vi "Predictor.vi"(9 "Measurement Cluster":T1, 10 "Peak Max Threshold":dbl=0.1 format="%#_13g", 11 "Data Cluster in":T3 {"Julabo Serial Configuration"."Flow Control" items=["None", "XON/XOFF", "RTS/CTS", "XON/XOFF & RTS/CTS", "DTR/DSR", "XON/XOFF & DTR/DSR"]; "Julabo Serial Configuration"."Stop Bits" items=["1.0"=10, "1.5"=15, "2.0"=20]; "Julabo Serial Configuration"."Data Bits" items=["7"=7, "8"=8]; "Julabo Serial Configuration"."Parity" items=["None", "Odd", "Even", "Mark", "Space"]; "Julabo Serial Configuration"."Baud Rate" items=["300"=300, "600"=600, "1200"=1200, "2400"=2400, "4800"=4800, "9600"=9600, "19200"=19200]; "XpU (0.6K) Ext" min=0.1 max=99.9; "Tv (0s) Ext" max=999; "Tn (3s) Ext" min=3 max=9999; "Xp (0.6K) Ext" min=0.1 max=99.9; "Tv (0s) Int" max=999; "Tn (3s) Int" min=3 max=9999; "Xp (0.6K) Int" min=0.1 max=99.9; "Lower Bandlimit" min=0.0 max=200.0; "Upper Bandlimit" min=0.0 max=200.0; "InternMin" format="%.2f"; "InternMax" format="%.2f"; "CoolMax" min=-100 max=0; "HeatMax" max=100; "Subtemp" format="%.2f"; "Overtemp" format="%.2f"; "Julabo Setpoint" format="%.2f"; "Current DoE" format="%0.3f"}) -> (3 "Data Cluster out":T3 {"Julabo Serial Configuration"."Flow Control" items=["None", "XON/XOFF", "RTS/CTS", "XON/XOFF & RTS/CTS", "DTR/DSR", "XON/XOFF & DTR/DSR"]; "Julabo Serial Configuration"."Stop Bits" items=["1.0"=10, "1.5"=15, "2.0"=20]; "Julabo Serial Configuration"."Data Bits" items=["7"=7, "8"=8]; "Julabo Serial Configuration"."Parity" items=["None", "Odd", "Even", "Mark", "Space"]; "Julabo Serial Configuration"."Baud Rate" items=["300"=300, "600"=600, "1200"=1200, "2400"=2400, "4800"=4800, "9600"=9600, "19200"=19200]; "XpU (0.6K) Ext" min=0.1 max=99.9; "Tv (0s) Ext" max=999; "Tn (3s) Ext" min=3 max=9999; "Xp (0.6K) Ext" min=0.1 max=99.9; "Tv (0s) Int" max=999; "Tn (3s) Int" min=3 max=9999; "Xp (0.6K) Int" min=0.1 max=99.9; "Lower Bandlimit" min=0.0 max=200.0; "Upper Bandlimit" min=0.0 max=200.0; "InternMin" format="%.2f"; "InternMax" format="%.2f"; "CoolMax" min=-100 max=0; "HeatMax" max=100; "Subtemp" format="%.2f"; "Overtemp" format="%.2f"; "Julabo Setpoint" format="%.2f"; "Current DoE" format="%0.3f"})   [LabVIEW 2015]
uses:
  --Controls and TypeDefs--/DoE_Control_Cluster.ctl
  <instrlib>/JULABO DeviceDriver/Examples/Julabo Serial Control.ctl
  --Controls and TypeDefs--/Measurement_Cluster.ctl
  --Controls and TypeDefs--/Raman_Model_Data_Cluster.ctl
panel:
  # "Flow Rate Measurements"
  # "Temp Measurements"
  # "Raman Measurements"
  # "Julabo"
  # "Limits"
  # "PID Control Parameters"
  # "Julabo"
  # "Limits"
  # "PID Control Parameters"
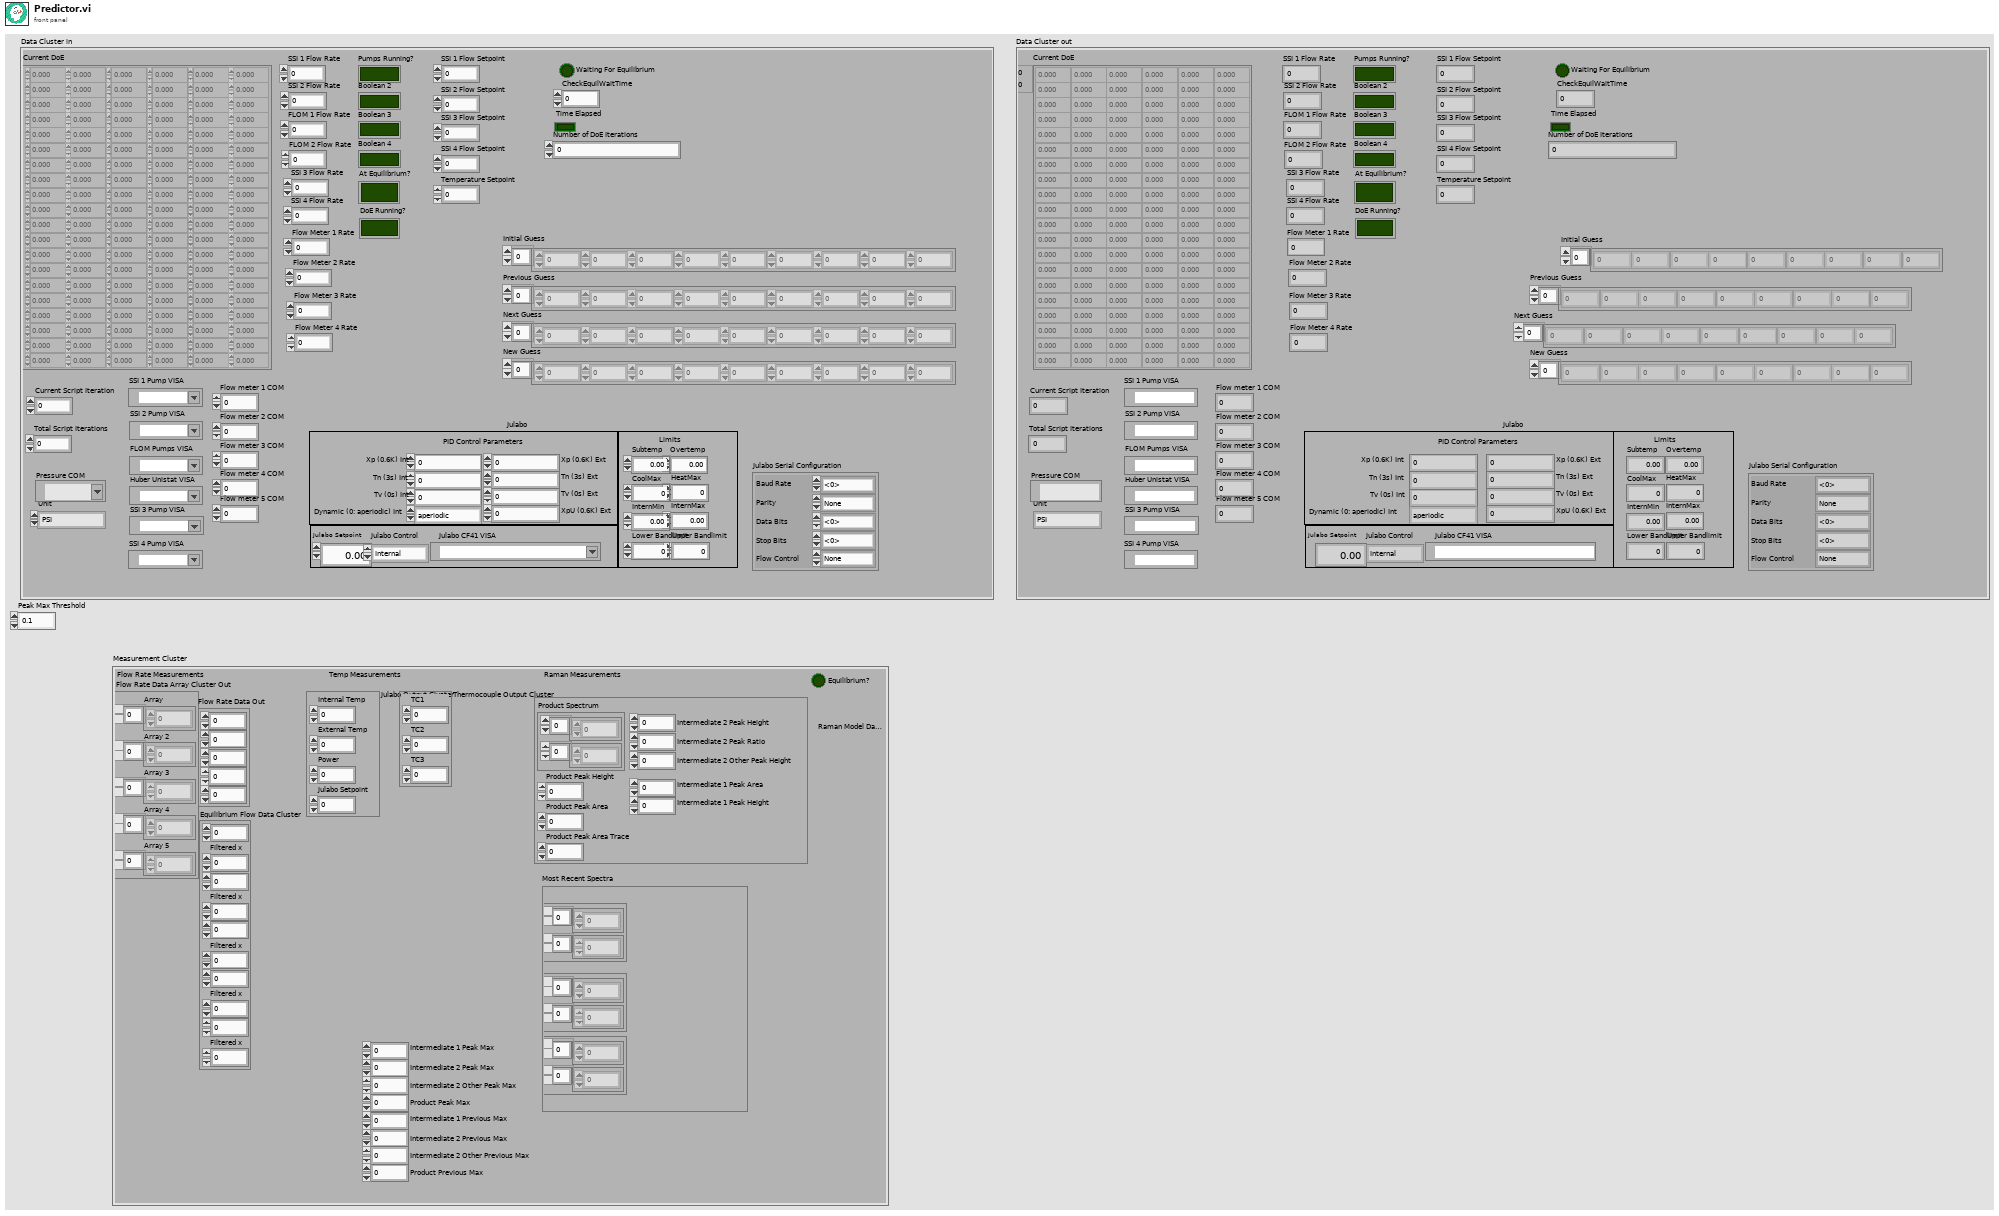
[diagram p1: front panel]
types:
  T1 = typedef "Measurement_Cluster.ctl" = cluster{"Raman Model Data Cluster":T2, "Julabo Output Cluster":cluster{"Internal Temp":dbl, "External Temp":dbl, "Power":i8, "Julabo Setpoint":dbl}, "Thermocouple Output Cluster":cluster{"TC1":dbl, "TC2":dbl, "TC3":dbl}, "Flow Rate Data Array Cluster Out":cluster{"Array":dbl[], "Array 2":dbl[], "Array 3":dbl[], "Array 4":dbl[], "Array 5":dbl[]}, "Flow Rate Data Out":cluster{dbl, dbl, dbl, dbl, dbl}, "Equilibrium?":bool, "Equilibrium Flow Data Cluster":cluster{dbl, "Filtered x":dbl, dbl, "Filtered x":dbl, dbl, "Filtered x":dbl, dbl, "Filtered x":dbl, dbl, "Filtered x":dbl}, "Most Recent Spectra":cluster{"Most recent Channel 3 (Intermediate 1) Spectrum":cluster{i32[], i32[]}, "Most recent Channel 2 (Intermediate 2) Spectrum":cluster{i32[], i32[]}, "Most recent Channel 1 (Product) Spectrum":cluster{i32[], i32[]}}, "Intermediate 2 Other Peak Max":i32, "Intermediate 2 Peak Max":i32, "Intermediate 1 Peak Max":i32, "Product Peak Max":i32, "Intermediate 2 Other Previous Max":i32, "Intermediate 2 Previous Max":i32, "Intermediate 1 Previous Max":i32, "Product Previous Max":i32}
  T2 = typedef "Raman_Model_Data_Cluster.ctl" = cluster{"Product Spectrum":cluster{i32[], i32[]}, "Product Peak Height":i32, "Product Peak Area":i32, "Product Peak Area Trace":i32, "Intermediate 2 Peak Height":i32, "Intermediate 1 Peak Area":i32, "Intermediate 1 Peak Height":i32, "Intermediate 2 Other Peak Height":i32, "Intermediate 2 Peak Ratio":i32}
  T3 = typedef "DoE_Control_Cluster.ctl" = cluster{"Current DoE":dbl[][], "SSI 1 Flow Rate":dbl, "SSI 2 Flow Rate":dbl, "FLOM 1 Flow Rate":dbl, "FLOM 2 Flow Rate":dbl, "Pumps Running?":bool, "Boolean 2":bool, "Boolean 3":bool, "Boolean 4":bool, "At Equilibrium?":bool, "DoE Running?":bool, "Current Script Iteration":dbl, "Total Script Iterations":dbl, "FLOM Pumps VISA":refnum<visa-resource-name>, "SSI 1 Pump VISA":refnum<visa-resource-name>, "SSI 2 Pump VISA":refnum<visa-resource-name>, "Huber Unistat VISA":refnum<visa-resource-name>, "SSI 3 Pump VISA":refnum<visa-resource-name>, "SSI 4 Pump VISA":refnum<visa-resource-name>, "SSI 4 Flow Rate":dbl, "SSI 3 Flow Rate":dbl, "Flow Meter 1 Rate ":dbl, "Flow Meter 2 Rate":dbl, "Flow Meter 3 Rate":dbl, "Flow Meter 4 Rate":dbl, "SSI 1 Flow Setpoint":dbl, "SSI 2 Flow Setpoint":dbl, "SSI 3 Flow Setpoint":dbl, "SSI 4 Flow Setpoint":dbl, "Temperature Setpoint":dbl, "Flow meter 3 COM":u16, "Flow meter 5 COM":u16, "Flow meter 4 COM":u16, "Flow meter 2 COM":u16, "Flow meter 1 COM":u16, "Unit":enum16{"PSI", "Bar", "cm H2O", "ft H2O", "hectoPascal", "in Hg", "in H2O", "kiloPascal", "milliBar", "mmHg", "MegaPascal", "Numeric Pressure"}, "Pressure COM":refnum<visa-resource-name>, "Julabo Setpoint":dbl, "Julabo Control":enum16{"Internal", "External"}, "Overtemp":dbl, "Subtemp":dbl, "HeatMax":u8, "CoolMax":i8, "InternMax":dbl, "InternMin":dbl, "Upper Bandlimit":dbl, "Lower Bandlimit":dbl, "Julabo CF41 VISA":refnum<visa-resource-name>, "Xp (0.6K) Int":dbl, "Tn (3s) Int":u16, "Tv (0s) Int":u16, "Dynamic (0: aperiodic) Int":enum16{"aperiodic", "standard"}, "Xp (0.6K) Ext":dbl, "Tn (3s) Ext":u16, "Tv (0s) Ext":u16, "XpU (0.6K) Ext":dbl, "Julabo Serial Configuration":T4, "Waiting For Equilibrium":bool, "CheckEquilWaitTime":dbl, "Time Elapsed":bool, "Initial Guess":dbl[], "Next Guess":dbl[], "Previous Guess":dbl[], "Number of DoE Iterations":i32, "New Guess":dbl[]}
  T4 = typedef "Julabo Serial Control.ctl" = cluster{"Baud Rate":u32, "Parity":u16, "Data Bits":u16, "Stop Bits":u16, "Flow Control":u16}
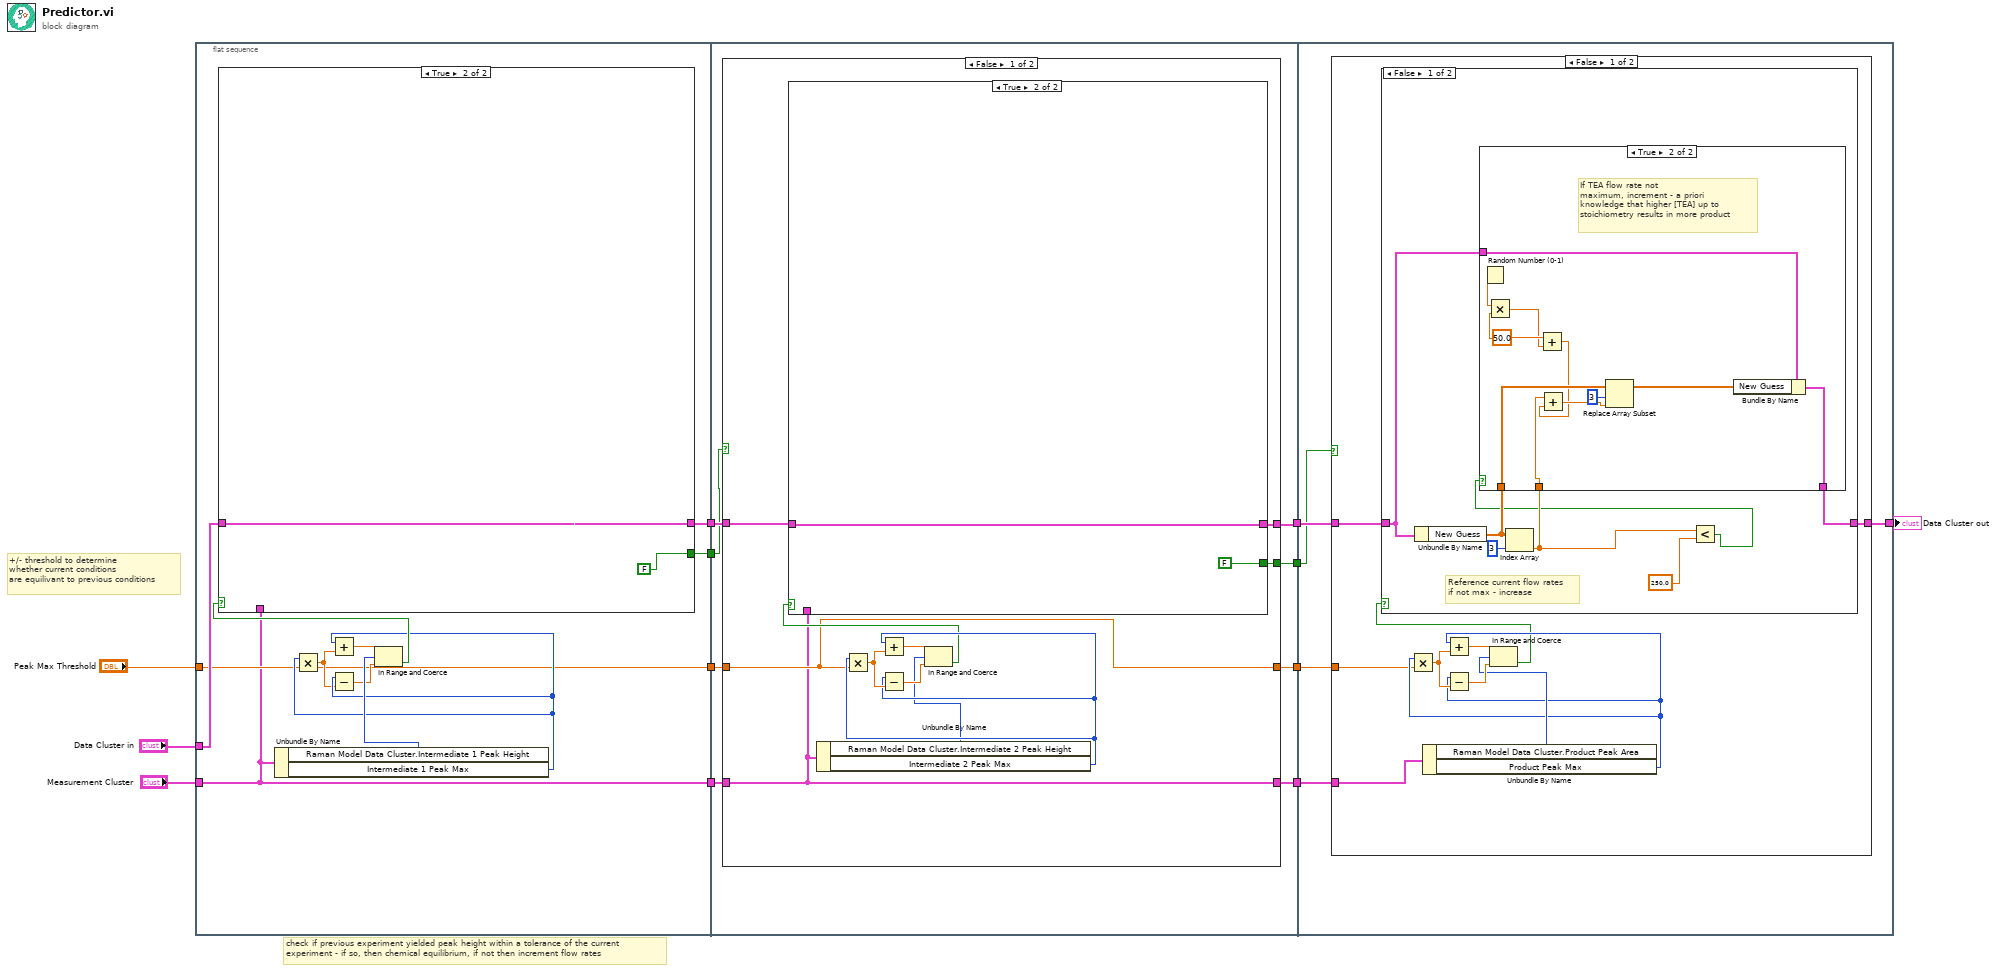
[diagram p0: block diagram]
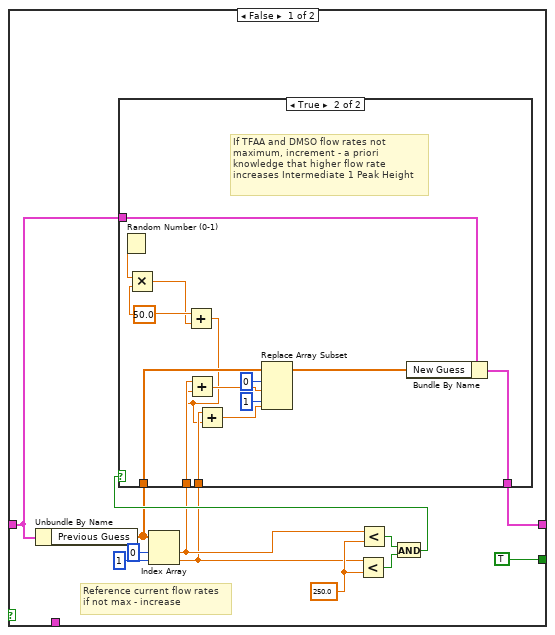
[diagram p2: hidden frame]
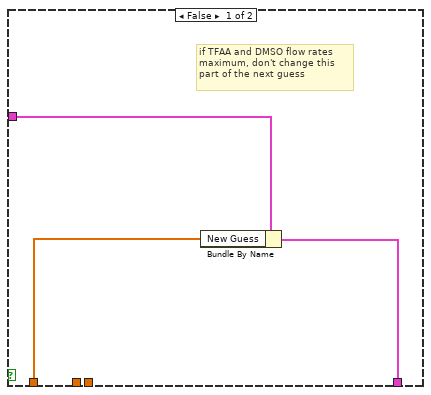
[diagram p3: hidden frame]
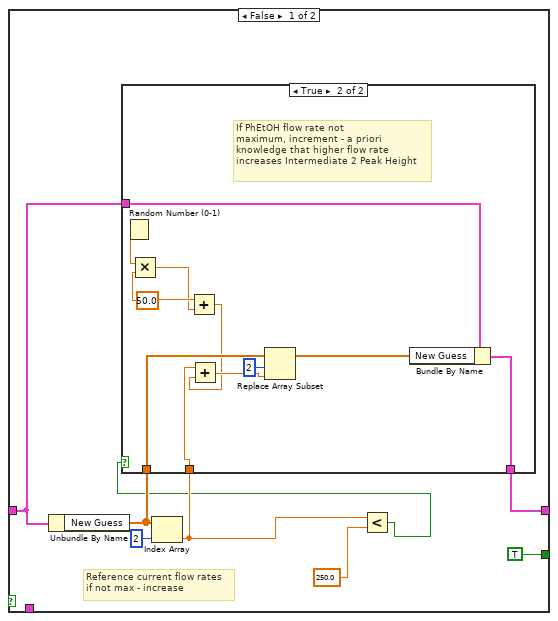
[diagram p4: hidden frame]
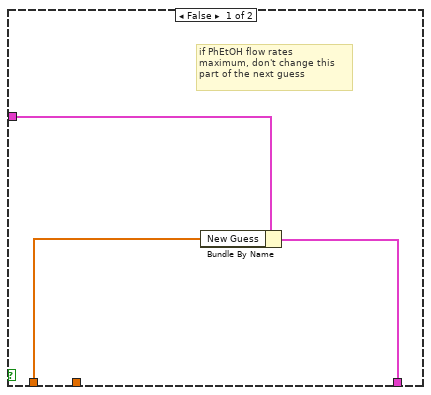
[diagram p5: hidden frame]
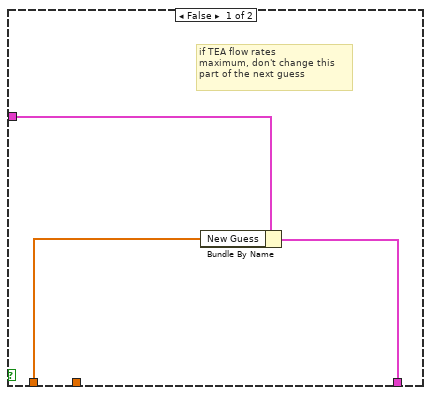
[diagram p7: hidden frame]
diagram:
  # "check if previous experiment yielded peak height within a tolerance of the current\nexperiment - if so, then chemical equilibrium, if not then increment flow rates"
  # "+/- threshold to determine\nwhether current conditions\nare equilivant to previous conditions"
  n1 = flat-sequence {
    tunnel: [w23] -> w12
    tunnel: "Data Cluster in" -> [w21]
    tunnel: "Measurement Cluster" -> [w14]
    tunnel: [w14] -> w7
    tunnel: "Peak Max Threshold" -> [w15]
    tunnel: [w15] -> w4
    tunnel: [w13] -> w3
    tunnel: w12 -> [w61]
    tunnel: [w59] -> w11
    tunnel: w7 -> [w60]
    tunnel: [w57] -> w6
    tunnel: w4 -> [w62]
    tunnel: w3 -> [w56]
    tunnel: [w58] -> w2
    tunnel: [w55] -> w1
    tunnel: w11 -> [w104]
    tunnel: [w103] -> w10
    tunnel: w6 -> [w105]
    tunnel: w2 -> [w106]
    tunnel: w1 -> [w102]
    frame #0 {
      n2 = Unbundle By Name(w14) -> ("Raman Model Data Cluster.Intermediate 1 Peak Height"=w20:i32, "Intermediate 1 Peak Max"=w19:i32)
      n3 = Multiply(x=w19, y=w15) -> (x*y=w18:dbl)
      n4 = Add(x=w19, y=w18) -> (x+y=w17:dbl)
      n5 = Subtract(x=w19, y=w18) -> (x-y=w16:dbl)
      n6 = In Range and Coerce(upper limit=w17, x=w20, lower limit=w16) -> (In Range?=w22:bool)  [unwired: 1 out]
      n7 = case shown="True" w22 {
        tunnel: [w25 w54] -> w23
        tunnel: w21 -> [w29 w54]
        tunnel: w14 -> [_ _]
        tunnel: [TRUE FALSE] -> w13
        frame False {
          w32 = 250.0 ("y")
          # "Reference current flow rates\nif not max - increase"
          n8 = Unbundle By Name(w29) -> ("Previous Guess"=w28:dbl[])
          n9 = Index Array(array=w28, index #1=0 ("index"), index #2=1 ("index")) -> (element #1=w27:dbl, element #2=w26:dbl)
          n10 = Less?(x=w26, y=w32) -> (x < y?=w33:bool)
          n11 = Less?(x=w27, y=w32) -> (x < y?=w34:bool)
          n12 = And(x=w34, y=w33) -> (x .and. y?=w35:bool)
          n13 = case shown="True" w35 {
            tunnel: w29 -> [w38 w51]
            tunnel: w28 -> [w36 w52]
            tunnel: w27 -> [_ w48]
            tunnel: w26 -> [_ w47]
            tunnel: [w37 w43] -> w25
            frame False {
              # "if TFAA and DMSO flow rates\nmaximum, don't change this\npart of the next guess"
              n14 = Bundle By Name(cluster=w38, "New Guess"=w36) -> (w37:T3)
            }
            frame True {
              w41 = 50.0 ("y")
              # "If TFAA and DMSO flow rates not\nmaximum, increment - a priori\nknowledge that higher flow rate\nincreases Intermediate 1 Peak Height"
              n15 = Random Number (0-1)() -> (number: 0 to 1=w42:dbl)
              n16 = Multiply(x=w42, y=w41) -> (x*y=w40:dbl)
              n17 = Add(x=w41, y=w40) -> (x+y=w39:dbl)
              n18 = Add(x=w48, y=w39) -> (x+y=w46:dbl)
              n19 = Add(x=w47, y=w39) -> (x+y=w45:dbl)
              n20 = Replace Array Subset(array=w52, new element #1=w46, index #1=0 ("index"), new element #2=w45, index #2=1 ("index")) -> (w44:dbl[])
              n21 = Bundle By Name(cluster=w51, "New Guess"=w44) -> (w43:T3)
            }
          }
        }
        frame True {
        }
      }
    }
    frame #1 {
      n22 = case shown="False" w56 {
        selector: w56 -> [_ w98]
        tunnel: w62 -> [w65 w101]
        tunnel: w61 -> [w68 w100]
        tunnel: w60 -> [w64 w99]
        tunnel: [w67 w100] -> w59
        tunnel: [w65 w101] -> w58
        tunnel: [w64 w99] -> w57
        tunnel: [w63 w98] -> w55
        frame False {
          n23 = Unbundle By Name(w64) -> ("Raman Model Data Cluster.Intermediate 2 Peak Height"=w69:i32, "Intermediate 2 Peak Max"=w70:i32)
          n24 = Multiply(x=w70, y=w65) -> (x*y=w73:dbl)
          n25 = Add(x=w70, y=w73) -> (x+y=w72:dbl)
          n26 = Subtract(x=w70, y=w73) -> (x-y=w71:dbl)
          n27 = In Range and Coerce(upper limit=w72, x=w69, lower limit=w71) -> (In Range?=w66:bool)  [unwired: 1 out]
          n28 = case shown="True" w66 {
            tunnel: [w76 w97] -> w67
            tunnel: w68 -> [w79 w97]
            tunnel: w64 -> [_ _]
            tunnel: [TRUE FALSE] -> w63
            frame False {
              # "Reference current flow rates\nif not max - increase"
              n29 = Unbundle By Name(w79) -> ("New Guess"=w78:dbl[])
              n30 = Index Array(array=w78, index=2) -> (element=w77:dbl)
              n31 = Less?(x=w77, y=250.0) -> (x < y?=w75:bool)
              n32 = case shown="True" w75 {
                tunnel: w79 -> [w84 w94]
                tunnel: w78 -> [w82 w95]
                tunnel: w77 -> [_ w92]
                tunnel: [w83 w89] -> w76
                frame False {
                  # "if PhEtOH flow rates\nmaximum, don't change this\npart of the next guess"
                  n33 = Bundle By Name(cluster=w84, "New Guess"=w82) -> (w83:T3)
                }
                frame True {
                  w87 = 50.0 ("y")
                  # "If PhEtOH flow rate not\nmaximum, increment - a priori\nknowledge that higher flow rate\nincreases Intermediate 2 Peak Height"
                  n34 = Random Number (0-1)() -> (number: 0 to 1=w88:dbl)
                  n35 = Multiply(x=w88, y=w87) -> (x*y=w86:dbl)
                  n36 = Add(x=w87, y=w86) -> (x+y=w85:dbl)
                  n37 = Add(x=w92, y=w85) -> (x+y=w91:dbl)
                  n38 = Replace Array Subset(array=w95, new element=w91, index=2) -> (w90:dbl[])
                  n39 = Bundle By Name(cluster=w94, "New Guess"=w90) -> (w89:T3)
                }
              }
            }
            frame True {
            }
          }
        }
        frame True {
        }
      }
    }
    frame #2 {
      n40 = case shown="False" w102 {
        tunnel: w106 -> [w111 _]
        tunnel: w105 -> [w110 _]
        tunnel: w104 -> [w109 w139]
        tunnel: [w108 w139] -> w103
        frame False {
          n41 = Unbundle By Name(w110) -> ("Raman Model Data Cluster.Product Peak Area"=w113:i32, "Product Peak Max"=w112:i32)
          n42 = Multiply(x=w112, y=w111) -> (x*y=w116:dbl)
          n43 = Add(x=w112, y=w116) -> (x+y=w115:dbl)
          n44 = Subtract(x=w112, y=w116) -> (x-y=w114:dbl)
          n45 = In Range and Coerce(upper limit=w115, x=w113, lower limit=w114) -> (In Range?=w107:bool)  [unwired: 1 out]
          n46 = case shown="False" w107 {
            tunnel: [w118 w138] -> w108
            tunnel: w109 -> [w121 w138]
            frame False {
              # "Reference current flow rates\nif not max - increase"
              n47 = Unbundle By Name(w121) -> ("New Guess"=w120:dbl[])
              n48 = Index Array(array=w120, index=3) -> (element=w119:dbl)
              n49 = Less?(x=w119, y=250.0) -> (x < y?=w117:bool)
              n50 = case shown="True" w117 {
                tunnel: w121 -> [w126 w136]
                tunnel: w120 -> [w124 w137]
                tunnel: w119 -> [_ w134]
                tunnel: [w125 w131] -> w118
                frame False {
                  # "if TEA flow rates\nmaximum, don't change this\npart of the next guess"
                  n51 = Bundle By Name(cluster=w126, "New Guess"=w124) -> (w125:T3)
                }
                frame True {
                  w129 = 50.0 ("y")
                  # "If TEA flow rate not\nmaximum, increment - a priori\nknowledge that higher [TEA] up to \nstoichiometry results in more product"
                  n52 = Random Number (0-1)() -> (number: 0 to 1=w130:dbl)
                  n53 = Multiply(x=w130, y=w129) -> (x*y=w128:dbl)
                  n54 = Add(x=w129, y=w128) -> (x+y=w127:dbl)
                  n55 = Add(x=w134, y=w127) -> (x+y=w133:dbl)
                  n56 = Replace Array Subset(array=w137, new element=w133, index=3) -> (w132:dbl[])
                  n57 = Bundle By Name(cluster=w136, "New Guess"=w132) -> (w131:T3)
                }
              }
            }
            frame True {
            }
          }
        }
        frame True {
        }
      }
    }
  }
  "Data Cluster out" <- w10
